vi "Stop Module.vi"(8 "error in (no error)":errorcluster, 9 "Wait for Module to stop? (F)":bool, 10 "Origin":string, 11 "Module ID":i32=-1) -> (0 "error out":errorcluster)   [LabVIEW 2020, in "TCP Client.lvlib"]
doc: "Send the Stop request to the Module's Main.vi. If <b>Wait for Module to stop?</b> is TRUE, then this VI will not complete execution until the Module Main VI has stopped running.\n\n<b>Note:</b> If the cloneable module is running as singleton, then the 'Wait for Module to stop?' input is ignored... this VI will <b>always</b> wait until a cloneable Main VI running as singleton has stopped running.\n_____\nBased on Delacor QMH Project Template 6.0.0.89."
uses:
  TCP Client.lvlib
  Stop Argument--cluster.ctl
  Module Running State--enum.ctl
  <vilib>/event_ctls.llb/usereventprio.ctl
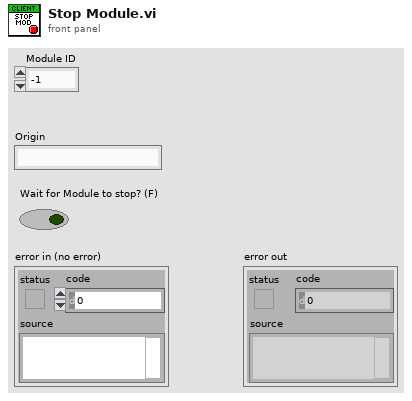
[diagram p1: front panel]
types:
  T1 = typedef "TCP Client.lvlib/Module Running State--enum.ctl" = enum16{"Not Running", "Running as Cloneable", "Running as Singleton"}
  T2 = typedef "TCP Client.lvlib/Stop Argument--cluster.ctl" = cluster{"Module ID":i32, "Origin":string, "Exit via Stop Module Req?":bool, "Wait for Module to stop?":bool}
  T3 = typedef "TCP Client.lvlib/Request Events--cluster.ctl" = cluster{"Stop Module":refnum<user-event>, "Show Panel":refnum<user-event>, "Hide Panel":refnum<user-event>, "Show Diagram":refnum<user-event>, "Get Module Execution Status":refnum<user-event>, "Connect to TCP Server":refnum<user-event>}
  T4 = typedef "usereventprio.ctl" = enum32{"high priority", "normal priority"}
  T5 = enum32{"Bad", "Idle", "Run top level", "Running"}
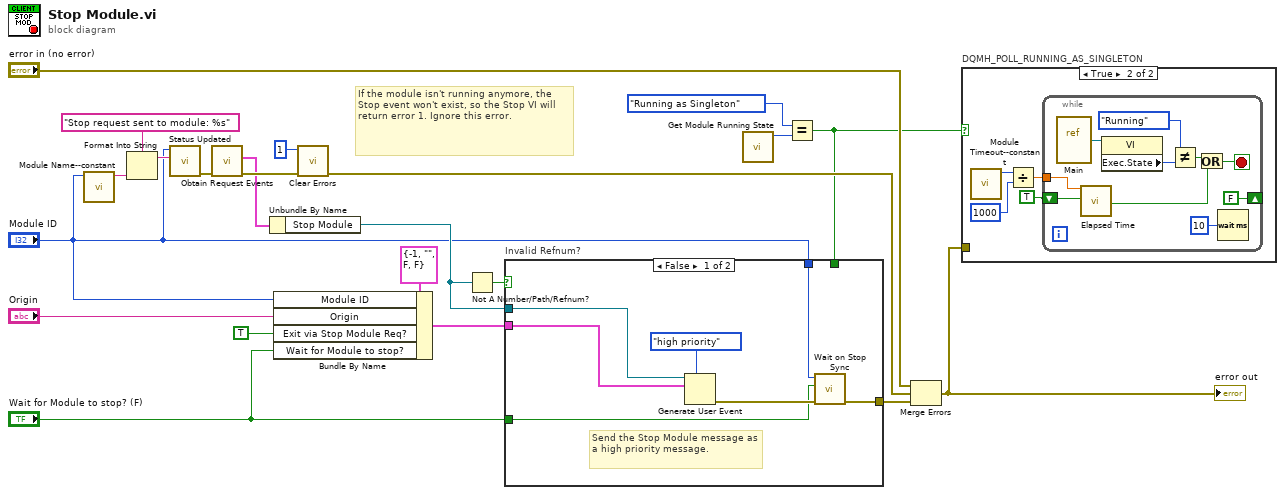
[diagram p0: block diagram]
diagram:
  # "If the module isn't running anymore, the Stop event won't exist, so the Stop VI will return error 1. Ignore this error."
  n1 = call "Module Name--constant.vi"("Module ID"="Module ID") -> ("Module Name"=w19:string)  [unwired: 10 in]
  n2 = Format Into String(format string="Stop request sent to module: %s", w19) -> (resulting string=w20:string)  [unwired: 2 in, 1 out]
  n3 = call "Status Updated.vi"("Status"=w20, "Module ID"="Module ID") -> ("error out"=w13:errorcluster)  [unwired: 9 in]
  n4 = call "Obtain Request Events.vi"("error in (no error)"=w13) -> ("error out"=w12:errorcluster, "TCP Client Request Events"=w10:T3)  [unwired: 9 in]
  n5 = Unbundle By Name(w10) -> ("Stop Module"=w15:refnum<user-event>)
  n6 = Bundle By Name(cluster=T2 {"Module ID"=-1, "Origin"="", "Exit via Stop Module Req?"=FALSE, "Wait for Module to stop?"=FALSE} ("event data"), "Module ID"="Module ID", "Origin"="Origin", "Exit via Stop Module Req?"=TRUE, "Wait for Module to stop?"="Wait for Module to stop? (F)") -> (w14:T2)
  n7 = call <vilib>:"Clear Errors.vi"("error in (no error)"=w12, "specific error code to clear (0: all)"=1) -> ("error out"=w9:errorcluster)  [unwired: 4 in, 1 out]
  n8 = Not A Number/Path/Refnum?(number/path/refnum=w15) -> (NaN/Path/Refnum?=w16:bool)
  n9 = call "Get Module Running State.vi"() -> ("Module Running State"=w4:T1)  [unwired: 11 in]
  n10 = Equal?(x=Module_Running_State--enum."Running as Singleton", y=w4) -> (x = y?=w3:bool)
  n11 = case "Invalid Refnum?" shown="False" w16 {
    tunnel: [w25 _] -> w8
    tunnel: w14 -> [w29 _]
    tunnel: w15 -> [w28 _]
    tunnel: "Module ID" -> [w24 _]
    tunnel: "Wait for Module to stop? (F)" -> [w23 _]
    tunnel: w3 -> [_ _]
    frame False {
      # "Send the Stop Module message as a high priority message."
      n12 = Generate User Event(priority (normal)=usereventprio."high priority", user event=w28, event data cluster=w29) -> (error out=w26:errorcluster)  [unwired: 1 in, 1 out]
      n13 = call "Wait on Stop Sync.vi"("error in (no error)"=w26, "Wait for Module to stop?"=w23, "Module ID"=w24) -> ("error out"=w25:errorcluster)  [unwired: 8 in]
    }
    frame True {
      # "Module is exiting. No need to send the standard \"not running\" error that is sent in other request VIs."
    }
  }
  n14 = Merge Errors("error in (no error)", w9, w8) -> (w1:errorcluster)
  "error out" <- w1
  n15 = case "DQMH_POLL_RUNNING_AS_SINGLETON" shown="True" w3 {
    tunnel: w1 -> [_ _]
    frame False {
    }
    frame True {
      n16 = call "Module Timeout--constant.vi"() -> ("Module Timeout"=w33:i32)  [unwired: 11 in]
      n17 = Divide(x=w33, y=1000) -> (x/y=w31:dbl)
      n18 = while {
        tunnel: w31 -> [w36]
        shift-right: [FALSE] -> _
        shift-left: TRUE -> [w37]
        stop <- w39 stop-if-true
        n19 = vi-ref "Main.vi"() -> (w43:refnum<vi>)
        n20 = call "Elapsed Time"("Time Target (s)"=w36, "Reset"=w37) -> ("Time has Elapsed"=w35:bool)  [unwired: 10 in, 7 out]
        n21 = property class="VI"(reference=w43) -> ("Exec.State"=w42:T5)  [unwired: 1 in, 2 out]
        n22 = Not Equal?(x=T5."Running", y=w42) -> (x != y?=w40:bool)
        n23 = Or(x=w40, y=w35) -> (x .or. y?=w39:bool)
        n24 = Wait (ms)(milliseconds to wait=u32 10) -> ()  [unwired: 1 out]
      }
    }
  }
